vi "Generate RPC Methods.vi"(7 "RPC Method Parameters":T1[](array[typedef]), 8 "error in (no error)":errorcluster, 10 "Library":refnum<vi>, 11 "Server class in":refnum<vi>) -> (0 "error out":errorcluster, 3 "Server class out":refnum<vi>)   [LabVIEW 2019, in "gRPC Template Creation Utility.lvlib"]
uses:
  gRPC Template Creation Utility.lvlib
  TypeDefs/RPC Method Parameters.ctl
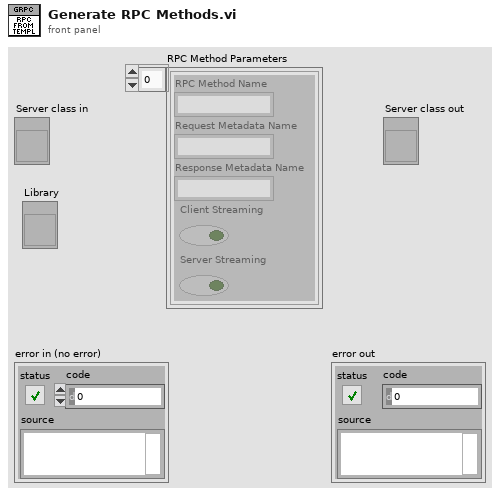
[diagram p1: front panel]
types:
  T1 = typedef "gRPC Template Creation Utility.lvlib/RPC Method Parameters.ctl" = cluster{"RPC Method Name":string, "Request Metadata Name":string, "Response Metadata Name":string, "Client Streaming":bool, "Server Streaming":bool}
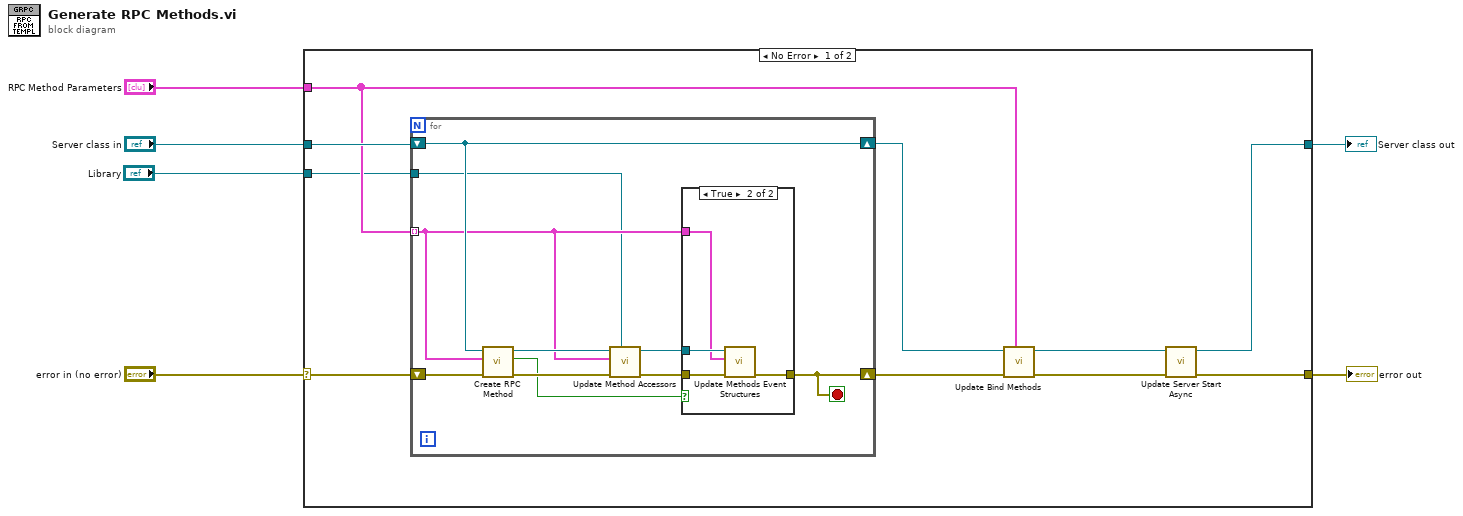
[diagram p0: block diagram]
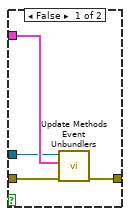
[diagram p2: hidden frame]
diagram:
  n1 = case shown="No Error" "error in (no error)" {
    selector: "error in (no error)" -> [w16 w36]
    tunnel: [w10 w36] -> w6
    tunnel: "Server class in" -> [w15 w35]
    tunnel: [w8 w35] -> w3
    tunnel: "RPC Method Parameters" -> [w13 _]
    tunnel: "Library" -> [w7 _]
    frame No Error {
      n2 = for {
        tunnel: w13 -> [w19] mode=indexing
        shift-right: [w25] -> w14
        shift-left: w16 -> [w26]
        shift-right: [w24] -> w12
        shift-left: w15 -> [w24]
        tunnel: w7 -> [w17]
        stop <- w25 stop-if-true
        n3 = call "Create RPC Method.vi"("error in (no error)"=w26, "RPC Method Parameters"=w19, "Server class in"=w24) -> ("error out"=w21:errorcluster, "Newly created ?"=w18:bool, "Server class out"=w23:refnum<vi>)  [unwired: 6 in]
        n4 = call "Update Method Accessors.vi"("Library"=w17, "error in (no error)"=w21, "RPC Method Parameters"=w19, "Server class in"=w23) -> ("error out"=w20:errorcluster, "Server class out"=w22:refnum<vi>)  [unwired: 6 in]
        n5 = case shown="True" w18 {
          tunnel: w20 -> [w30 w34]
          tunnel: w22 -> [w27 w33]
          tunnel: w19 -> [w28 w32]
          tunnel: [w29 w31] -> w25
          frame False {
            n6 = call "Update Methods Event Unbundlers.vi"("error in (no error)"=w30, "RPC Method Parameters"=w28, "LVClassLibrary in"=w27) -> ("error out"=w29:errorcluster)  [unwired: 7 in, 1 out]
          }
          frame True {
            n7 = call "Update Methods Event Structures.vi"("error in (no error)"=w34, "RPC Method Parameters"=w32, "LVClassLibrary in"=w33) -> ("error out"=w31:errorcluster)  [unwired: 7 in, 1 out]
          }
        }
      }
      n8 = call "Update Bind Methods.vi"("RPC Method Parameters"=w13, "error in (no error)"=w14, "Server class in"=w12) -> ("error out"=w11:errorcluster, "Server class out"=w9:refnum<vi>)  [unwired: 7 in]
      n9 = call "Update Server Start Async.vi"("error in (no error)"=w11, "Server class in"=w9) -> ("error out"=w10:errorcluster, "Server class out"=w8:refnum<vi>)  [unwired: 8 in]
    }
    frame Error {
    }
  }
  "error out" <- w6
  "Server class out" <- w3
